vi "Returning Values By Reference Array Of Complex Struct.vi"(10 "length":i32, 11 "triangles":T1) -> (2 "name":string, 3 "triangles out":T1)   [LabVIEW 2018, in "ParsingDataSampleDLL.lvlib"]
doc: "__declspec(dllexport) void ReturningValuesByReference_ArrayOfComplexStruct (struct complexStructPolygon **triangles, int length);"
uses:
  <vilib>/Utility/importsl/GetValueByPointer/datatype.ctl
  <vilib>/Utility/importsl/GetValueByPointer/GetValueByPointer.xnode
  ParsingDataSampleDLL.lvlib
  ni_reference_vs/Debug/ParsingDataSampleDLL.dll
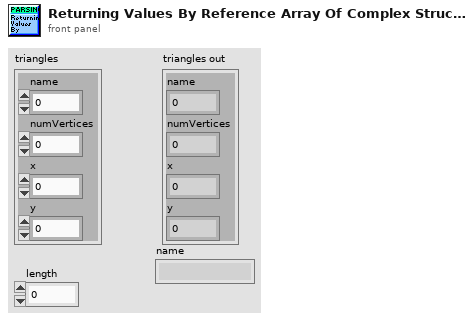
[diagram p1: front panel]
types:
  T1 = cluster{"name":u32, "numVertices":i32, "x":i32, "y":i32}
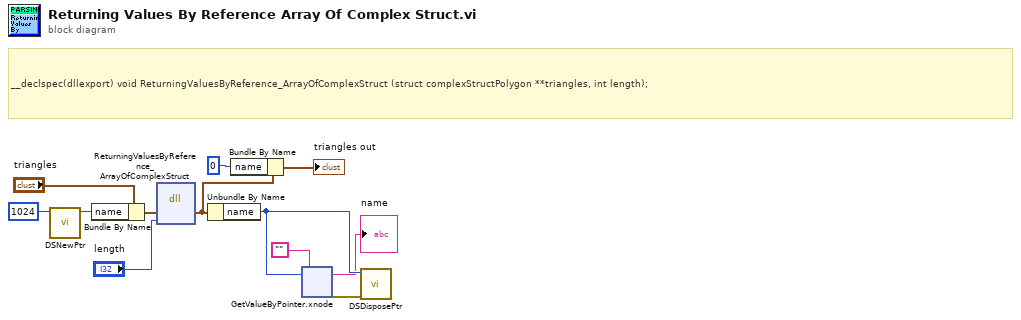
[diagram p0: block diagram]
diagram:
  # "__declspec(dllexport) void ReturningValuesByReference_ArrayOfComplexStruct (struct complexStructPolygon **triangles, int length);"
  n1 = call <vilib>:"DSNewPtr.vi"("Size"=u64 1024) -> ("Pointer"=w10:u64)  [unwired: 9 in, 1 out]
  n2 = Bundle By Name(cluster="triangles", "name"=w10) -> (w9:T1)
  n3 = dll-call lib="C:/Users/celit/Documents/GitHub/Labview_Python_DLL_Call/ni_reference_vs/Debug/ParsingDataSampleDLL.*" fn="ReturningValuesByReference_ArrayOfComplexStruct"("triangles"=w9, "length"="length") -> ("triangles"=w4:T1)  [unwired: 5 in, 2 out]
  n4 = Unbundle By Name(w4) -> ("name"=w7:u32)
  n5 = Bundle By Name(cluster=w4, "name"=u32 0) -> (→"triangles out":T1)
  n6 = xnode "GetValueByPointer.xnode"("Pointer"=w7, "InputType"="") -> ("Output"=→"name":string, "ErrorOut"=w8:errorcluster)  [unwired: 2 in]
  n7 = call <vilib>:"DSDisposePtr.vi"("error in (no error)"=w8, "Pointer"=w7) -> ()  [unwired: 9 in, 1 out]
